vi "Play with rts cts.vi"(8 "error in (no error)":errorcluster, 11 "Serial open? (y)":bool=TRUE) -> (0 "error out":errorcluster, 1 "RTS control ok?":bool, 3 "PassFail":string, 4 "Comport responsive?":bool, 5 "Comport unresponsive?":bool)   [LabVIEW 2013]
uses:
  NanoArduino/NanoCmds.ctl
  Test Globals/Global 1.vi
  Main Support/Global 2.vi
panel:
  in  "Modem port":refnum<visa-resource-name>="COM30"
  out "read buffer":string
  out "VISA resource name out":refnum<visa-resource-name>
  out "read buffer 3":string
  out "read buffer 2":string
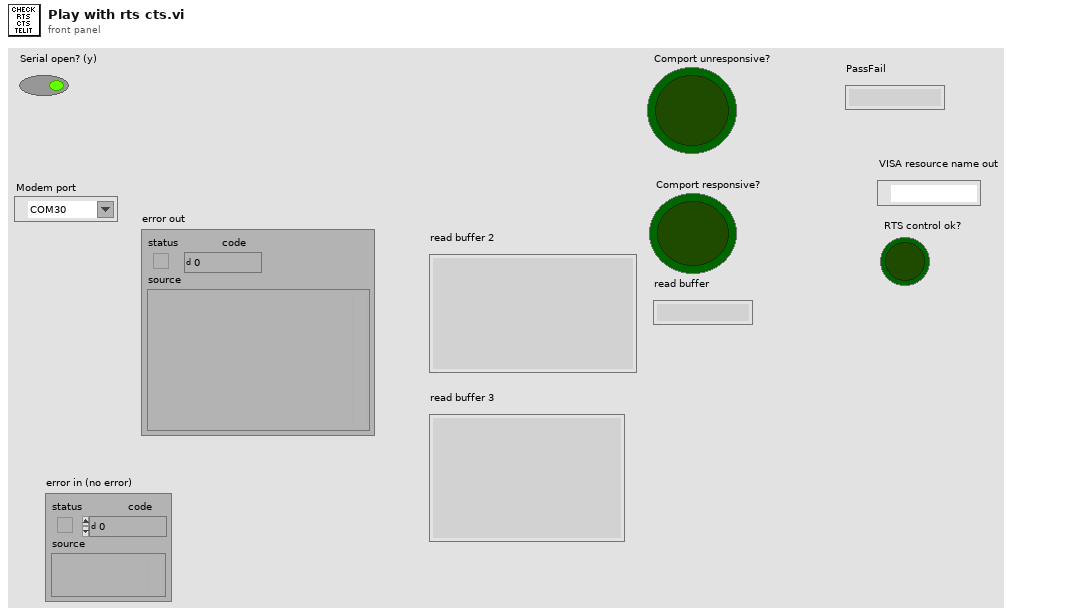
[diagram p1: front panel]
types:
  T1 = typedef "NanoCmds.ctl" = enum16{"Make digital port an output", "Make digital port an input", "Set digital pin high", "Set digital pin low", "Get digital pin state", "Get analog pin voltage", "Get analog pins difference", "Get ohms at analog pin", "Turn on current limit", "Reset Nano device", "Get digital pin state pullup", "Read current", "Initialize", "Power up uut", "Power down uut", "Get uut current draw", "Set ADC volts high", "Set ADC volts low", "Start up uut modem", "Get CTS state", "Get on_nsleep state", "Reset modem", "Get lid state", "Wait for lid closed", "Wait for lid open", "Power up, start, get curr", "Check if X2 shorted", "Power up and start up", "Check X3 shorted", "Get RTS state", "Get DTR state", "Reboot 1002759"}
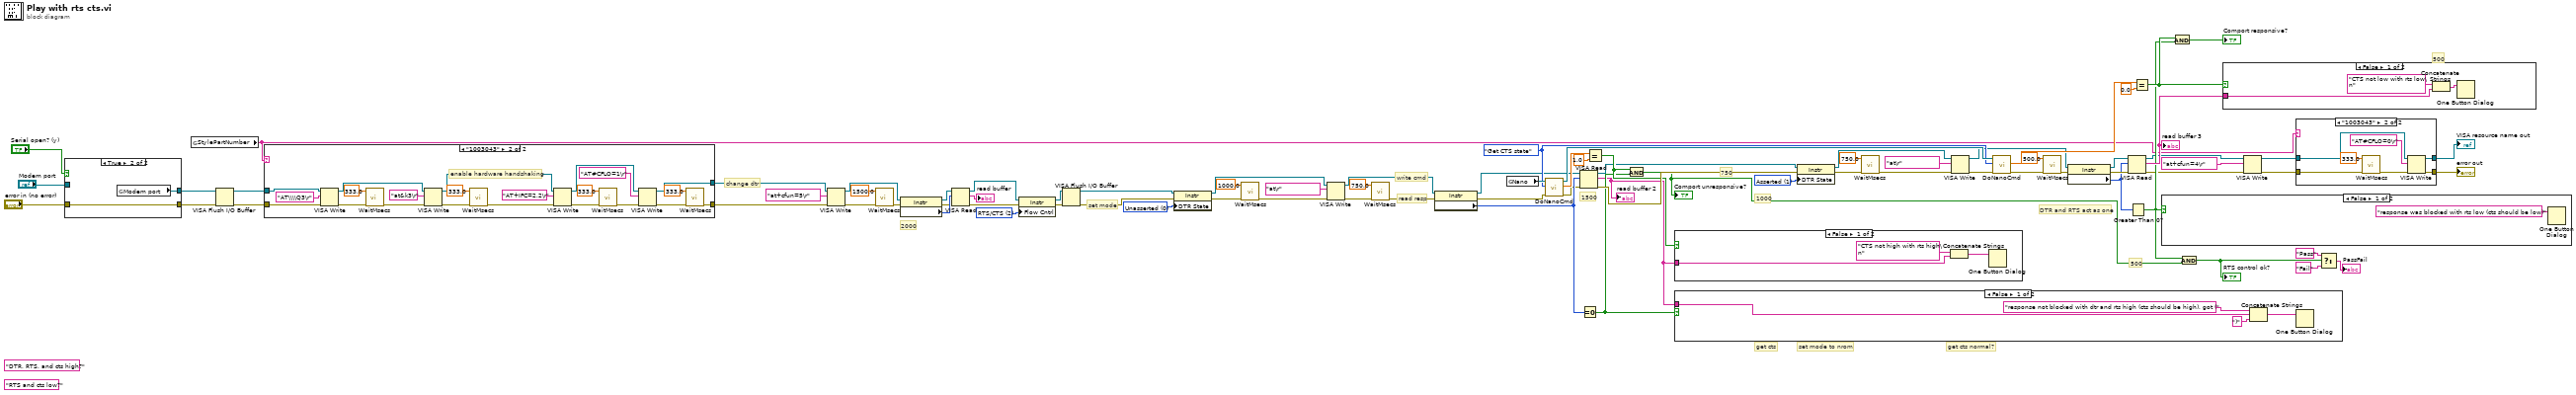
[diagram p0: block diagram]
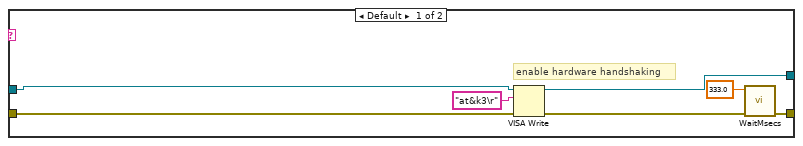
[diagram p3: hidden frame]
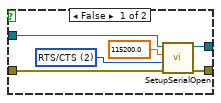
[diagram p4: hidden frame]
diagram:
  (unwired) "RTS and cts low?" ("Message")
  (unwired) "DTR, RTS, and cts high?" ("Message")
  w49 = u16 2 items=["None", "XON/XOFF", "RTS/CTS", "XON/XOFF & RTS/CTS", "DTR/DSR", "XON/XOFF & DTR/DSR"] ("Serial Settings:Flow Control")
  w55 = NanoCmds."Get CTS state" ("Nano Op")
  w77 = i16 1 items=["Unknown"=-1, "Unasserted"=0, "Asserted"=1] ("Serial Settings:Modem Line Settings:Line DTR State")
  w81 = i16 0 items=["Unknown"=-1, "Unasserted"=0, "Asserted"=1] ("Serial Settings:Modem Line Settings:Line DTR State")
  # "DTR and RTS act as one"
  # "500"
  # "500"
  # "750"
  # "1000"
  # "2000"
  # "1500"
  # "get cts normal?"
  # "set mode to nrom"
  # "read resp"
  # "get cts"
  # "write cmd"
  # "set mode"
  # "change dtr"
  n1 = case shown="True" "Serial open? (y)" {
    tunnel: [w84 w90] -> w10
    tunnel: "Modem port" -> [w88 _]
    tunnel: "error in (no error)" -> [w87 w89]
    tunnel: [w83 w89] -> w11
    frame False {
      w85 = u16 2 items=["None", "XON/XOFF", "RTS/CTS", "XON/XOFF & RTS/CTS", "DTR/DSR", "XON/XOFF & DTR/DSR"] ("flow control (0:none)")
      n2 = call "SetupSerialOpen.vi"("error in (no error)"=w87, "flow control (0:none)"=w85, "Baud"=115200.0, "VISA Refnum in"=w88) -> ("error out"=w83:errorcluster, "VISA session"=w84:refnum<visa-resource-name>)  [unwired: 6 in]
    }
    frame True {
      n3 = global read "Global 1.vi" "Modem port"() -> (w90:refnum<visa-resource-name>)
    }
  }
  n4 = global read "Global 2.vi" "StylePartNumber"() -> (w3:string)
  n5 = VISA Flush I/O Buffer(VISA resource name=w10, error in (no error)=w11) -> (VISA resource name out=w9:refnum<visa-resource-name>, error out=w8:errorcluster)  [unwired: 1 in]
  n6 = case shown="\"1003043\"" w3 {
    tunnel: w9 -> [w94 w116]
    tunnel: w8 -> [w93 w118]
    tunnel: [w92 w106] -> w7
    tunnel: [w91 w105] -> w6
    frame Default {
      # "enable hardware handshaking"
      n7 = VISA Write(VISA resource name=w94, write buffer="at&k3\r", error in (no error)=w93) -> (VISA resource name out=w91:refnum<visa-resource-name>, error out=w95:errorcluster)  [unwired: 1 out]
      n8 = call "WaitMsecs.vi"("error in (no error)"=w95, "Wait Msecs"=333.0) -> ("error out"=w92:errorcluster)  [unwired: 9 in]
    }
    frame "1003043" {
      # "enable hardware handshaking"
      n9 = VISA Write(VISA resource name=w116, write buffer="AT\\\\Q3\r", error in (no error)=w118) -> (VISA resource name out=w102:refnum<visa-resource-name>, error out=w115:errorcluster)  [unwired: 1 out]
      n10 = call "WaitMsecs.vi"("error in (no error)"=w115, "Wait Msecs"=333.0) -> ("error out"=w104:errorcluster)  [unwired: 9 in]
      n11 = VISA Write(VISA resource name=w102, write buffer="at&k3\r", error in (no error)=w104) -> (VISA resource name out=w101:refnum<visa-resource-name>, error out=w100:errorcluster)  [unwired: 1 out]
      n12 = call "WaitMsecs.vi"("error in (no error)"=w100, "Wait Msecs"=333.0) -> ("error out"=w98:errorcluster)  [unwired: 9 in]
      n13 = VISA Write(VISA resource name=w101, write buffer="AT+IFC=2,2\r", error in (no error)=w98) -> (VISA resource name out=w110:refnum<visa-resource-name>, error out=w112:errorcluster)  [unwired: 1 out]
      n14 = call "WaitMsecs.vi"("error in (no error)"=w112, "Wait Msecs"=333.0) -> ("error out"=w111:errorcluster)  [unwired: 9 in]
      n15 = VISA Write(VISA resource name=w110, write buffer="AT#CFLO=1\r", error in (no error)=w111) -> (VISA resource name out=w105:refnum<visa-resource-name>, error out=w107:errorcluster)  [unwired: 1 out]
      n16 = call "WaitMsecs.vi"("error in (no error)"=w107, "Wait Msecs"=333.0) -> ("error out"=w106:errorcluster)  [unwired: 9 in]
    }
  }
  n17 = VISA Write(VISA resource name=w6, write buffer="at+cfun=5\r", error in (no error)=w7) -> (VISA resource name out=w28:refnum<visa-resource-name>, error out=w32:errorcluster)  [unwired: 1 out]
  n18 = call "WaitMsecs.vi"("error in (no error)"=w32, "Wait Msecs"=1500.0) -> ("error out"=w27:errorcluster)  [unwired: 9 in]
  n19 = property class="Instr"(reference=w28, error in=w27) -> (reference out=w40:refnum<visa-resource-name>, error out=w39:errorcluster, "Serial Settings:Number of Bytes at Serial Port"=w41:u32)
  n20 = VISA Read(VISA resource name=w40, byte count=w41, error in (no error)=w39) -> (VISA resource name out=w31:refnum<visa-resource-name>, read buffer=→"read buffer":string, error out=w30:errorcluster)  [unwired: 1 out]
  n21 = property class="Instr"(reference=w31, error in=w30, "Flow Cntrl"=w49) -> (reference out=w44:refnum<visa-resource-name>, error out=w43:errorcluster)
  n22 = VISA Flush I/O Buffer(VISA resource name=w44, error in (no error)=w43) -> (VISA resource name out=w34:refnum<visa-resource-name>, error out=w33:errorcluster)  [unwired: 1 in]
  n23 = property class="Instr"(reference=w34, error in=w33, "DTR State"=w81) -> (reference out=w29:refnum<visa-resource-name>, error out=w25:errorcluster)
  n24 = call "WaitMsecs.vi"("error in (no error)"=w25, "Wait Msecs"=1000.0) -> ("error out"=w16:errorcluster)  [unwired: 9 in]
  n25 = VISA Write(VISA resource name=w29, write buffer="at\r", error in (no error)=w16) -> (VISA resource name out=w36:refnum<visa-resource-name>, error out=w48:errorcluster)  [unwired: 1 out]
  n26 = call "WaitMsecs.vi"("error in (no error)"=w48, "Wait Msecs"=750.0) -> ("error out"=w37:errorcluster)  [unwired: 9 in]
  n27 = property class="Instr"(reference=w36, error in=w37) -> (reference out=w54:refnum<visa-resource-name>, error out=w47:errorcluster, "Serial Settings:Number of Bytes at Serial Port"=w79:u32)
  n28 = global read "Global 1.vi" "Nano"() -> (w62:refnum<visa-resource-name>)
  n29 = call "DoNanoCmd.vi"("error in (no error)"=w47, "Nano Op"=w55, "VISA resource name"=w62) -> ("error out"=w46:errorcluster, "Read Value"=w61:dbl, "VISA resource name 2"=w59:refnum<visa-resource-name>)  [unwired: 5 in, 1 out]
  n30 = VISA Read(VISA resource name=w54, byte count=w79, error in (no error)=w46) -> (VISA resource name out=w53:refnum<visa-resource-name>, read buffer=w22:string, error out=w78:errorcluster)  [unwired: 1 out]
  "read buffer 2" <- w22
  n31 = Equal To 0?(x=w79) -> (x = 0?=w64:bool)
  n32 = Equal?(x=w61, y=1.0) -> (x = y?=w65:bool)
  n33 = And(x=w65, y=w64) -> (x .and. y?=w21:bool)
  "Comport unresponsive?" <- w21
  n34 = case shown="False" w65 {
    tunnel: w22 -> [w121 _]
    frame False {
      n35 = Concatenate Strings("CTS not high with rts high\n" ("message"), w121) -> (w120:string)
      n36 = One Button Dialog(message=w120) -> ()  [unwired: 1 in, 1 out]
    }
    frame True {
    }
  }
  n37 = case shown="False" w64 {
    tunnel: w22 -> [w125 _]
    frame False {
      n38 = Concatenate Strings("response not blocked with dtr and rts high (cts should be high), got (" ("message"), w125, ")" ("string")) -> (w123:string)
      n39 = One Button Dialog(message=w123) -> ()  [unwired: 1 in, 1 out]
    }
    frame True {
    }
  }
  n40 = property class="Instr"(reference=w53, error in=w78, "DTR State"=w77) -> (reference out=w52:refnum<visa-resource-name>, error out=w69:errorcluster)
  n41 = call "WaitMsecs.vi"("error in (no error)"=w69, "Wait Msecs"=750.0) -> ("error out"=w15:errorcluster)  [unwired: 9 in]
  n42 = VISA Write(VISA resource name=w52, write buffer="at\r", error in (no error)=w15) -> (VISA resource name out=w51:refnum<visa-resource-name>, error out=w58:errorcluster)  [unwired: 1 out]
  n43 = call "DoNanoCmd.vi"("error in (no error)"=w58, "Nano Op"=w55, "VISA resource name"=w59) -> ("error out"=w45:errorcluster, "Read Value"=w57:dbl)  [unwired: 5 in, 2 out]
  n44 = call "WaitMsecs.vi"("error in (no error)"=w45, "Wait Msecs"=500.0) -> ("error out"=w75:errorcluster)  [unwired: 9 in]
  n45 = property class="Instr"(reference=w51, error in=w75) -> (reference out=w50:refnum<visa-resource-name>, error out=w73:errorcluster, "Serial Settings:Number of Bytes at Serial Port"=w71:u32)
  n46 = VISA Read(VISA resource name=w50, byte count=w71, error in (no error)=w73) -> (VISA resource name out=w18:refnum<visa-resource-name>, read buffer=w35:string, error out=w17:errorcluster)  [unwired: 1 out]
  "read buffer 3" <- w35
  n47 = Greater Than 0?(x=w71) -> (x > 0?=w20:bool)
  n48 = Equal?(x=w57, y=0.0) -> (x = y?=w63:bool)
  n49 = case shown="False" w20 {
    frame False {
      n50 = One Button Dialog(message="response was blocked with rts low (cts should be low)") -> ()  [unwired: 1 in, 1 out]
    }
    frame True {
    }
  }
  n51 = And(x=w63, y=w20) -> (x .and. y?=→"Comport responsive?":bool)
  n52 = And(x=w20, y=w21) -> (x .and. y?=w19:bool)
  "RTS control ok?" <- w19
  n53 = case shown="False" w63 {
    tunnel: w35 -> [w129 _]
    frame False {
      n54 = Concatenate Strings("CTS not low with rts low\n" ("message"), w129) -> (w128:string)
      n55 = One Button Dialog(message=w128) -> ()  [unwired: 1 in, 1 out]
    }
    frame True {
    }
  }
  n56 = VISA Write(VISA resource name=w18, write buffer="at+cfun=4\r", error in (no error)=w17) -> (VISA resource name out=w4:refnum<visa-resource-name>, error out=w5:errorcluster)  [unwired: 1 out]
  n57 = case shown="\"1003043\"" w3 {
    tunnel: w4 -> [w131 w136]
    tunnel: w5 -> [w132 w137]
    tunnel: [w132 w134] -> w1
    tunnel: [w131 w133] -> w2
    frame Default {
    }
    frame "1003043" {
      n58 = call "WaitMsecs.vi"("error in (no error)"=w137, "Wait Msecs"=333.0) -> ("error out"=w138:errorcluster)  [unwired: 9 in]
      n59 = VISA Write(VISA resource name=w136, write buffer="AT#CFLO=0\r", error in (no error)=w138) -> (VISA resource name out=w133:refnum<visa-resource-name>, error out=w134:errorcluster)  [unwired: 1 out]
    }
  }
  "error out" <- w1
  "VISA resource name out" <- w2
  n60 = Select(t="Pass", s=w19, f="Fail") -> (s? t:f=→"PassFail":string)
